vi "ReadConfigKeys(Int32).vi"(0 "GRMActor in":refnum<class "GenericController.lvclass">, 5 "Config Refnum":T1, 7 "Keys":string[](array[string]), 9 "Default":i32[](array[numeric]), 11 "error in (no error)":errorcluster) -> (4 "GRMActor out":refnum<class "GenericController.lvclass">, 6 "Config Refnum dup":T1, 8 "Values":i32[](array[numeric]), 15 "error out":errorcluster)   [LabVIEW 2020, in "GenericController.lvlib" / "GenericController.lvclass"]
uses:
  GenericController.lvclass
  <vilib>/Utility/config.llb/Config Data RefNum.ctl
  <vilib>/Utility/config.llb/Read Key (I32).vi
  <vilib>/Utility/config.llb/Write Key (I32).vi
  <vilib>/Utility/config.llb/NI_LVConfig.lvlib
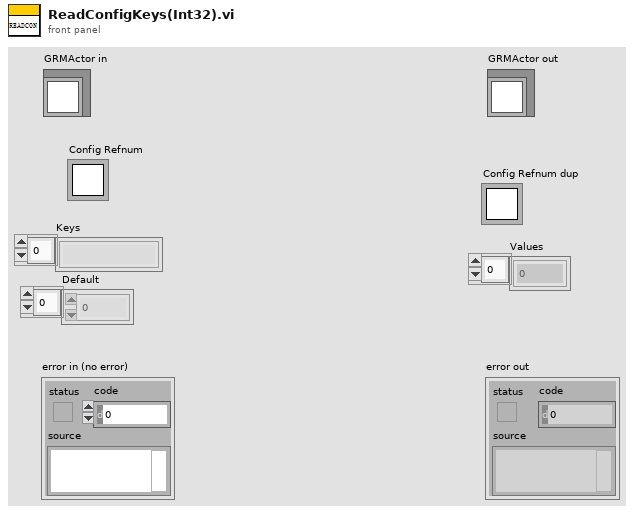
[diagram p1: front panel]
types:
  T1 = typedef "NI_LVConfig.lvlib/Config Data RefNum.ctl" = refnum<k1>
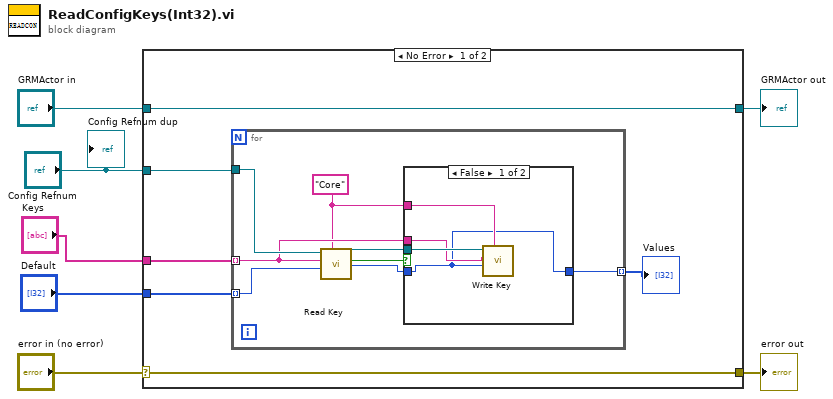
[diagram p0: block diagram]
diagram:
  n1 = case shown="No Error" "error in (no error)" {
    selector: "error in (no error)" -> [w12 w28]
    tunnel: [w12 w28] -> w6
    tunnel: [w13 w27] -> w4
    tunnel: "GRMActor in" -> [w13 w27]
    tunnel: "Config Refnum" -> [w11 _]
    tunnel: "Keys" -> [w10 _]
    tunnel: "Default" -> [w9 _]
    frame No Error {
      n2 = for {
        tunnel: w10 -> [w17] mode=indexing
        tunnel: w11 -> [w20]
        tunnel: w9 -> [w21] mode=indexing
        tunnel: [w14] -> w8 mode=indexing
        w15 = "Core" ("section")
        n3 = call-poly <vilib>:"Read Key.vi"("section"=w15, "default value"=w21, "key"=w17, "refnum"=w20) -> ("value"=w16:i32, "found?"=w19:bool, "refnum out"=w18:T1)  [unwired: 4 in, 1 out]
        n4 = case shown="False" w19 {
          tunnel: w18 -> [w25 _]
          tunnel: w17 -> [w24 _]
          tunnel: w16 -> [w22 w26]
          tunnel: w15 -> [w23 _]
          tunnel: [w22 w26] -> w14
          frame False {
            n5 = call-poly <vilib>:"Write Key.vi"("section"=w23, "value"=w22, "key"=w24, "refnum"=w25) -> ()  [unwired: 5 in, 3 out]
          }
          frame True {
          }
        }
      }
      "Values" <- w8
    }
    frame Error {
    }
  }
  "error out" <- w6
  "GRMActor out" <- w4
  "Config Refnum dup" <- "Config Refnum"
